vi "linear servo actuator.vi"() -> ()   [LabVIEW 2018]
panel:
  in  "Slide":dbl(slide) scale=0.0..10.0
  in  "stop":bool
  out "Waveform Chart":dynamicdata(graph) caption="Square"
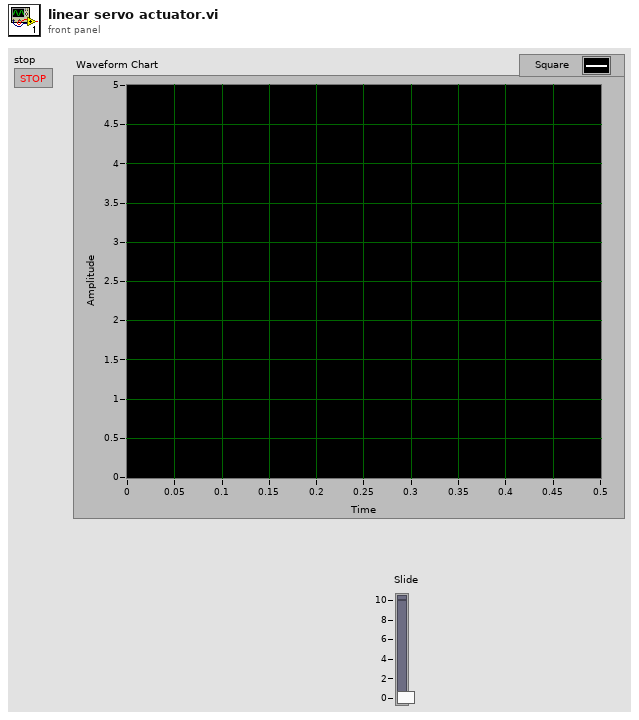
[diagram p1: front panel]
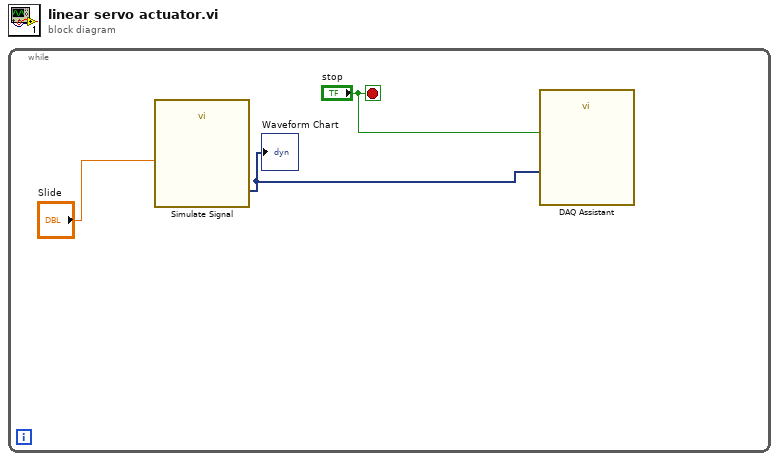
[diagram p0: block diagram]
diagram:
  n1 = while {
    stop <- "stop" stop-if-true
    n2 = call "Simulate Signal"("Duty Cycle (%)"="Slide") -> ("Square"=w3:dynamicdata)  [unwired: 13 in, 1 out]
    "Waveform Chart" <- w3
    n3 = call "DAQ Assistant"("data"=w3, "stop (F)"="stop") -> ()  [unwired: 15 in, 3 out]
  }
